vi "Agilent34410A Read.vi"(8 "error in (no error)":errorcluster, 11 "VISA Rsrc":refnum<visa-resource-name>="SR530") -> (0 "error out":errorcluster, 2 "Reading":dbl, 3 "VISA Rsrc Out":refnum<visa-resource-name>="GPIB0::12::INSTR", 4 "ChaineRep":string caption="Chaîne de commande")   [LabVIEW 2019]
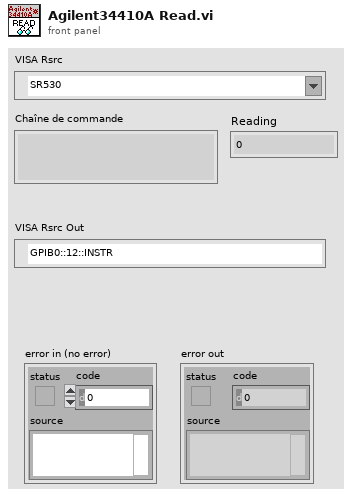
[diagram p1: front panel]
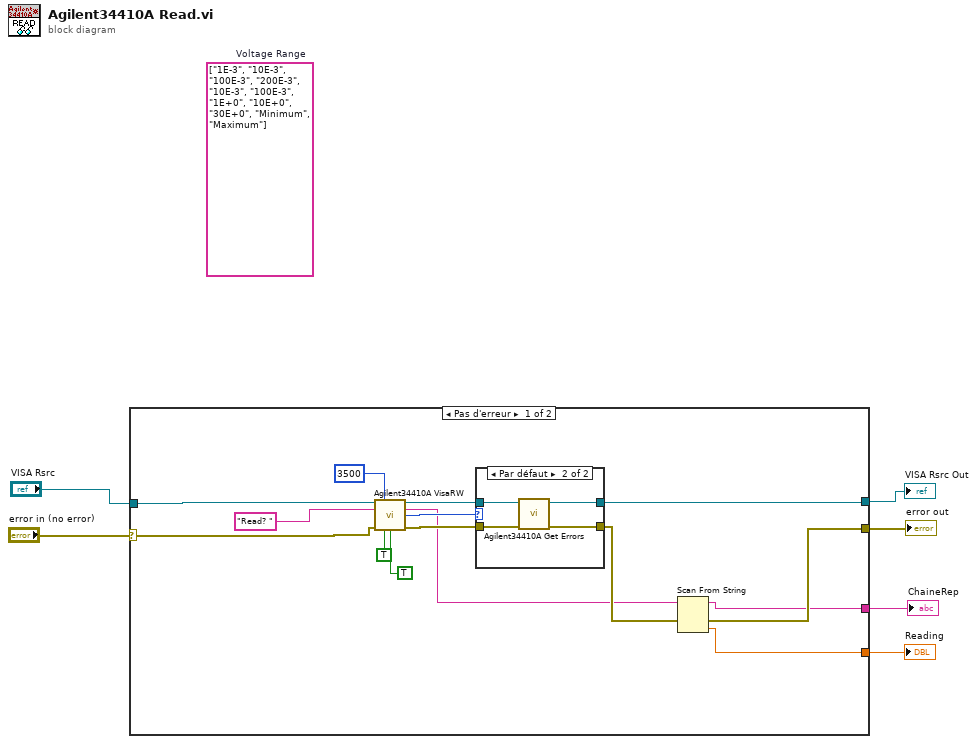
[diagram p0: block diagram]
diagram:
  (unwired) string[] ["1E-3", "10E-3", "100E-3", "200E-3", "10E-3", "100E-3", "1E+0", "10E+0", "30E+0", "Minimum", "Maximum"]  # Voltage Range
  n1 = case shown="Pas d'erreur" "error in (no error)" {
    selector: "error in (no error)" -> [w14 w28]
    tunnel: "VISA Rsrc" -> [w21 w29]
    tunnel: [w11 w28] -> w4
    tunnel: [w20 w29] -> w3
    tunnel: [w9 _] -> w2
    tunnel: [w8 _] -> w1
    frame No Error {
      n2 = call <userlib>:"Agilent34410A VisaRW.vi"("VISA Rsrc"=w21, "Timeout ms"=u32 3500, "ChaineCom"="Read? " ("string (\"\")"), "error in (no error)"=w14, "Lecture?(T)"=TRUE, "Poll?(F)"=TRUE) -> ("VISA Rsrc Out"=w18:refnum<visa-resource-name>, "ChaineRep"=w10:string, "octet d'état"=w17:u16, "error out"=w16:errorcluster)  [unwired: 5 in, 1 out]
      n3 = case shown="Par défaut" w17 {
        tunnel: w18 -> [w23 w27]
        tunnel: w16 -> [w22 w26]
        tunnel: [w22 w25] -> w12
        tunnel: [w23 w24] -> w20
        frame 0 {
        }
        frame Default {
          n4 = call <userlib>:"Agilent34410A Get Errors.vi"("error in (no error)"=w26, "VISA Rsrc"=w27) -> ("error out"=w25:errorcluster, "VISA Rsrc Out"=w24:refnum<visa-resource-name>)  [unwired: 7 in, 1 out]
        }
      }
      n5 = Scan From String(input string=w10, error in=w12) -> (remaining string=w9:string, error out=w11:errorcluster, output 1=w8:dbl)  [unwired: 3 in, 1 out]
    }
    frame Error {
    }
  }
  "error out" <- w4
  "VISA Rsrc Out" <- w3
  "ChaineRep" <- w2
  "Reading" <- w1
